vi "Pump_Data.vi"(8 "error in":errorcluster, 10 "Pump_data":T1 {"mix rpm" format="%.2f"; "Volume corrected" format="%.2f"; "Position_MM" format="%.3f"; "Volume PV" format="%.2f"; "Flow PV" format="%#.6f"; "Pressure PV" format="%.3f"}) -> (0 "error out":errorcluster)   [LabVIEW 2023, in "Drive.lvlib"]
doc: "_____\nCreated using DQMH Event Scripter 6.1.0.128."
uses:
  Drive.lvlib
  Pump_Data_Type.ctl
  Pump_Data Argument--cluster.ctl
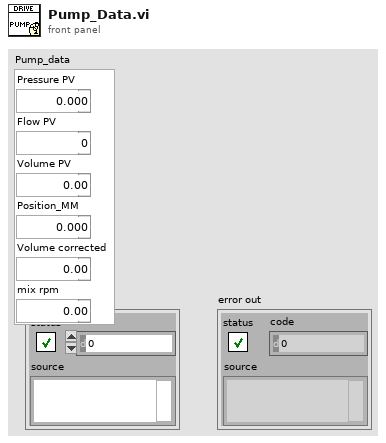
[diagram p1: front panel]
types:
  T1 = typedef "Drive.lvlib/Pump_Data_Type.ctl" = cluster{"Pressure PV":dbl, "Flow PV":dbl, "Volume PV":dbl, "Position_MM":dbl, "Volume corrected":dbl, "mix rpm":dbl}
  T2 = typedef "Drive.lvlib/Pump_Data Argument--cluster.ctl" = cluster{"Pump_data":T1}
  T3 = typedef "Drive.lvlib/Broadcast Events--cluster.ctl" = cluster{"Module Did Init":refnum<user-event>, "Status Updated":refnum<user-event>, "Error Reported":refnum<user-event>, "Module Did Stop":refnum<user-event>, "Update Module Execution Status":refnum<user-event>, "Pump_Data":refnum<user-event>, "Rotate Data":refnum<user-event>, "Pump2 data":refnum<user-event>}
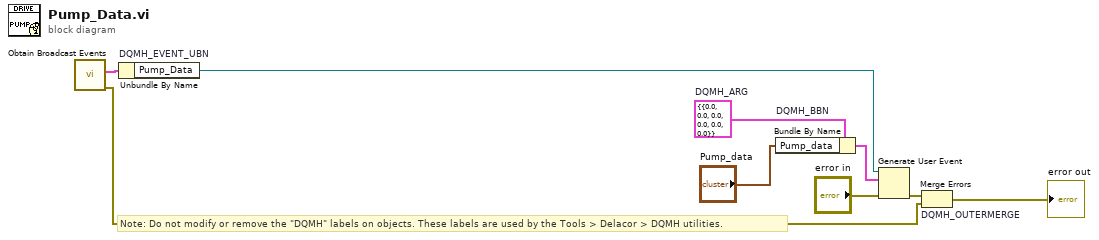
[diagram p0: block diagram]
diagram:
  w4 = T2 {"Pump_data"={"Pressure PV"=0.0, "Flow PV"=0.0, "Volume PV"=0.0, "Position_MM"=0.0, "Volume corrected"=0.0, "mix rpm"=0.0}}  # DQMH_ARG
  # "Note: Do not modify or remove the \"DQMH\" labels on objects. These labels are used by the Tools > Delacor > DQMH utilities."
  n1 = call "Obtain Broadcast Events.vi"() -> ("error out"=w2:errorcluster, "Drive Broadcast Events"=w1:T3)  [unwired: 10 in]
  n2 = Unbundle By Name "DQMH_EVENT_UBN"(w1) -> ("Pump_Data"=w6:refnum<user-event>)
  n3 = Bundle By Name "DQMH_BBN"(cluster=w4, "Pump_data"="Pump_data") -> (w7:T2)
  n4 = Generate User Event(user event=w6, event data cluster=w7, error in="error in") -> (error out=w5:errorcluster)  [unwired: 1 in, 1 out]
  n5 = Merge Errors "DQMH_OUTERMERGE"(w5, w2) -> (→"error out":errorcluster)
